vi "Launch Split Manager Tools Menu.vi"(8 "error in (no error)":errorcluster) -> (0 "error out":errorcluster)   [LabVIEW 2017]
doc: "This is a Tools Menu launcher for the Splitter Manager: \n\nhttps://forums.ni.com/t5/Quick-Drop-Enthusiasts/The-Splitter-amp-Pane-Manager/gpm-p/3834792\n\nEdited by Hooovahh"
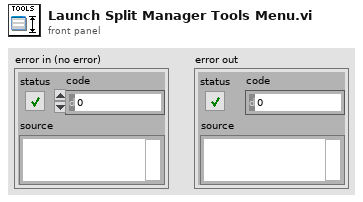
[diagram p1: front panel]
types:
  T1 = enum32{"Invalid", "Standard", "Closed", "Hidden", "Minimized", "Maximized"}
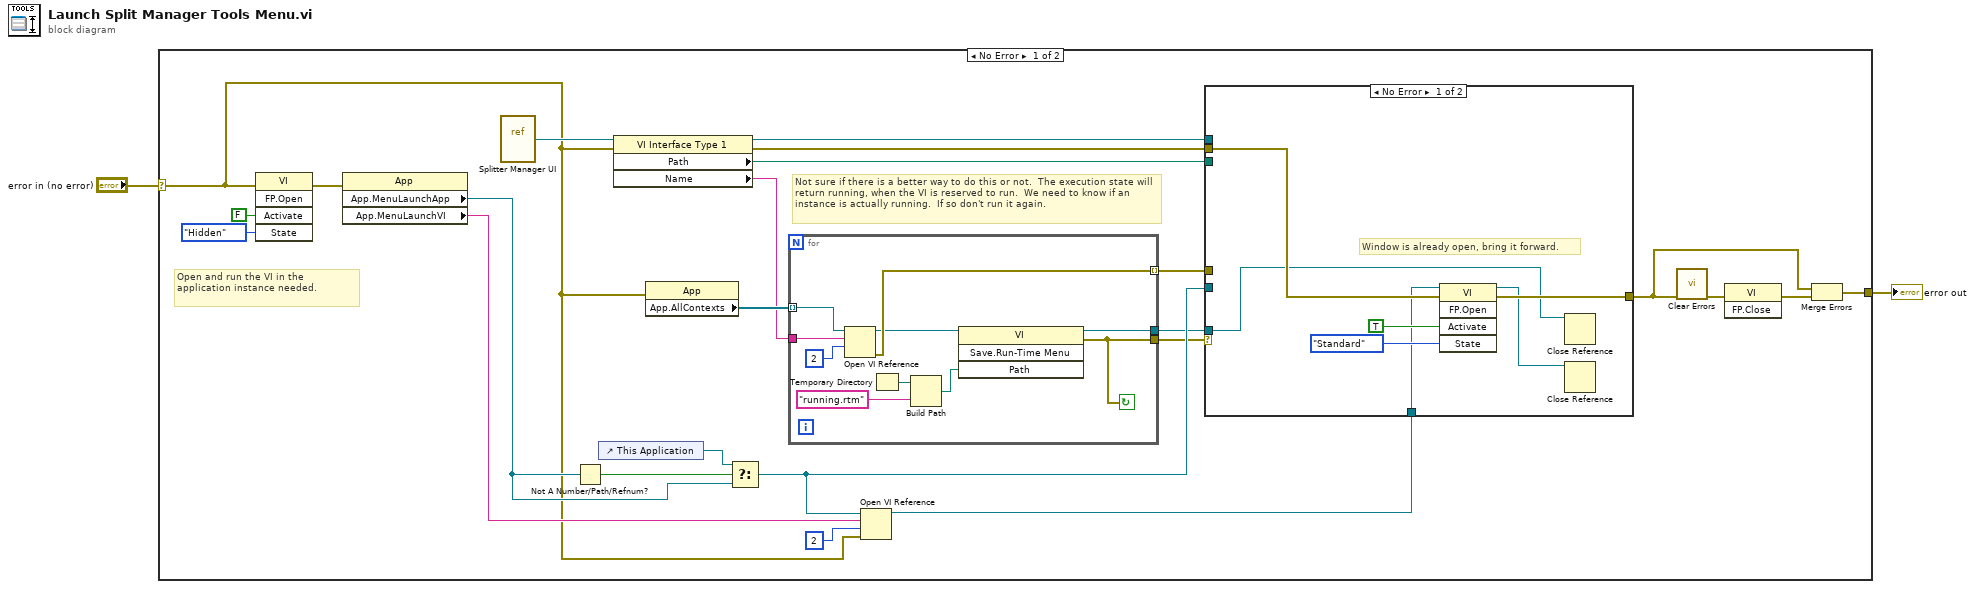
[diagram p0: block diagram]
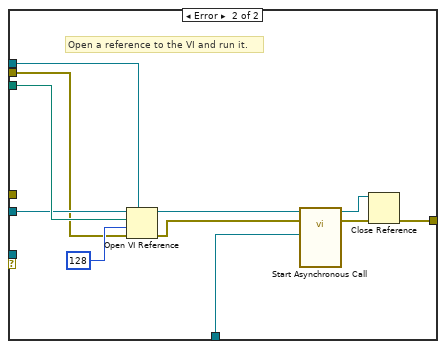
[diagram p2: hidden frame]
diagram:
  n1 = case shown="No Error" "error in (no error)" {
    selector: "error in (no error)" -> [w5 w55]
    tunnel: [w25 w55] -> w2
    frame No Error {
      # "Not sure if there is a better way to do this or not.  The execution state will return running, when the VI is reserved to run.  We need to know if an instance is actually running.  If so don't run it again."
      # "Open and run the VI in the application instance needed."
      n2 = invoke class="VI" method="FP.Open"(error in=w5, "Activate"=FALSE ("Activate?"), "State"=T1."Hidden") -> (error out=w15:errorcluster)  [unwired: 2 in, 4 out]
      n3 = property class="App"(error in=w15) -> ("App.MenuLaunchApp"=w19:refnum<vi>, "App.MenuLaunchVI"=w8:string)  [unwired: 1 in, 2 out]
      n4 = vi-ref "Splitter Manager UI.vi"() -> (w23:refnum<vi>)
      n5 = Not A Number/Path/Refnum?(number/path/refnum=w19) -> (NaN/Path/Refnum?=w21:bool)
      n6 = control-ref of="This Application"() -> (w20:refnum<vi>)
      n7 = property class="VI Interface Type 1"(reference=w23, error in=w5) -> (reference out=w11:refnum<vi>, error out=w18:errorcluster, "Path"=w22:path, "Name"=w12:string)
      n8 = property class="App"(error in=w5) -> ("App.AllContexts"=w13:refnum<vi>[])  [unwired: 1 in, 2 out]
      n9 = Select(t=w20, s=w21, f=w19) -> (s? t:f=w9:refnum<vi>)
      n10 = for {
        tunnel: w12 -> [w53]
        tunnel: w13 -> [w52] mode=indexing
        tunnel: [w46] -> w6
        tunnel: [w51] -> w4 mode=indexing
        tunnel: [w45] -> w3
        stop <- w46 continue-if-true
        n11 = Open VI Reference(application reference (local)=w52, vi path=w53, options=2) -> (vi reference=w47:refnum<vi>, error out=w51:errorcluster)  [unwired: 3 in]
        n12 = Temporary Directory() -> (w49:path)
        n13 = Build Path(base path=w49, name or relative path="running.rtm") -> (appended path=w50:path)
        n14 = invoke class="VI" method="Save.Run-Time Menu"(reference=w47, "Path"=w50) -> (reference out=w45:refnum<vi>, error out=w46:errorcluster)  [unwired: 2 in, 2 out]
      }
      n15 = Open VI Reference(application reference (local)=w9, vi path=w8, options=2, error in (no error)=w5) -> (vi reference=w7:refnum<vi>)  [unwired: 2 in, 1 out]
      n16 = case shown="No Error" w6 {
        tunnel: [w32 w44] -> w24
        tunnel: w22 -> [_ w43]
        tunnel: w9 -> [_ w41]
        tunnel: w18 -> [w33 w36]
        tunnel: w3 -> [w29 _]
        tunnel: w11 -> [_ w35]
        tunnel: w7 -> [w28 w34]
        tunnel: w4 -> [_ _]
        frame No Error {
          # "Window is already open, bring it forward."
          n17 = invoke class="VI" method="FP.Open"(reference=w28, error in=w33, "Activate"=TRUE ("Activate?"), "State"=T1."Standard") -> (reference out=w27:refnum<vi>, error out=w32:errorcluster)  [unwired: 1 in, 3 out]
          n18 = Close Reference(reference=w29) -> ()  [unwired: 1 in, 1 out]
          n19 = Close Reference(reference=w27) -> ()  [unwired: 1 in, 1 out]
        }
        frame Error {
          # "Open a reference to the VI and run it."
          n20 = Open VI Reference(type specifier VI Refnum (for type only)=w35, application reference (local)=w41, vi path=w43, options=128, error in (no error)=w36) -> (vi reference=w40:refnum<vi>, error out=w39:errorcluster)  [unwired: 1 in]
          n21 = call-by-ref "Start Asynchronous Call"(reference=w40, error in=w39, "VI Reference"=w34) -> (reference out=w37:refnum<vi>, error out=w38:errorcluster)  [unwired: 10 in, 1 out]
          n22 = Close Reference(reference=w37, error in (no error)=w38) -> (error out=w44:errorcluster)
        }
      }
      n23 = call <vilib>:"Clear Errors.vi"("error in (no error)"=w24) -> ("error out"=w26:errorcluster)  [unwired: 5 in, 1 out]
      n24 = invoke class="VI" method="FP.Close"(error in=w26) -> (error out=w14:errorcluster)  [unwired: 2 in, 2 out]
      n25 = Merge Errors(w24, w14) -> (w25:errorcluster)
    }
    frame Error {
    }
  }
  "error out" <- w2
